vi "Close.vi"(8 "error in":errorcluster, 10 "Data":variant) -> (0 "error out":errorcluster)   [LabVIEW 2010, in "Sensor Console.lvlib"]
doc: "This VI enqueues the named action."
uses:
  Sensor Console.lvlib
  Private Controls/Sensor Action.ctl
  Private Controls/Sensor Data Cluster.ctl
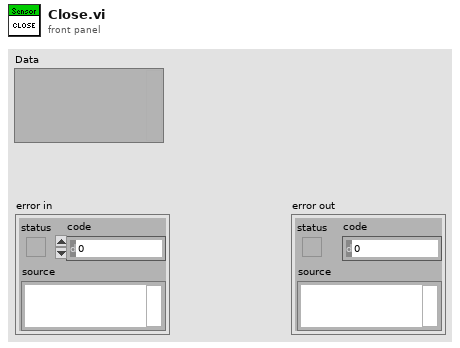
[diagram p1: front panel]
types:
  T1 = typedef "Sensor Console.lvlib/Sensor Data Cluster.ctl" = cluster{"Data":variant, "Action":T2}
  T2 = typedef "Sensor Console.lvlib/Sensor Action.ctl" = enum16{"Init", "Deposit", "Disburse", "Error", "Exit"}
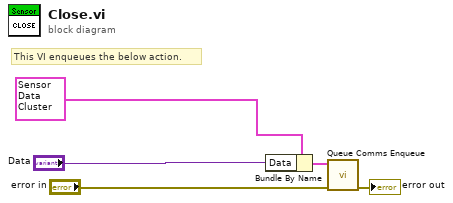
[diagram p0: block diagram]
diagram:
  # "This VI enqueues the below action."
  n1 = Bundle By Name(cluster=T1 {"Data"=variant, "Action"=enum."Exit"} ("element"), "Data"="Data") -> (w2:T1)
  n2 = call "Queue Comms Enqueue.vi"("error in"="error in", "element"=w2) -> ("error out"=→"error out":errorcluster)  [unwired: 9 in]
